vi "ENPH354_LabSCPE_(SubVI).vi"(10 "Save Data":path, 11 "Array":dbl[][](array[numeric])) -> (0 "I_sc [A]":dbl, 1 "I_m [A]":dbl, 2 "V_oc [V]":dbl, 3 "V_m [V]":dbl, 4 "FF":dbl, 5 "R_sh [Ohm]":dbl, 6 "PCE(n)":dbl, 7 "R_s [Ohm]":dbl)   [LabVIEW 2020]
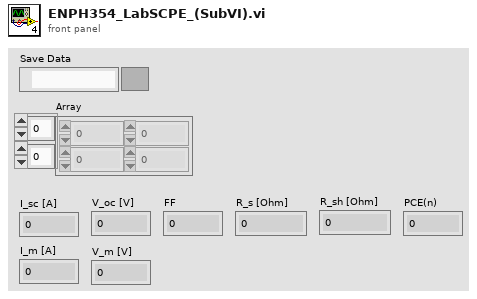
[diagram p1: front panel]
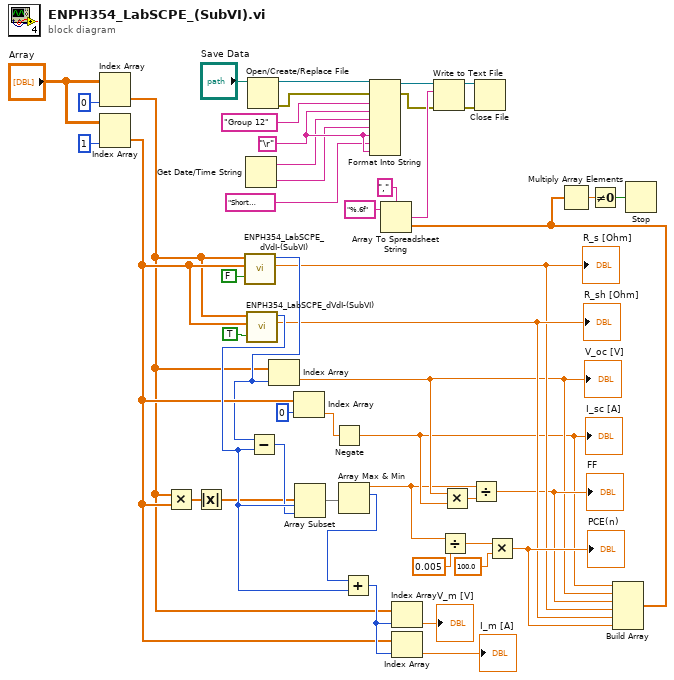
[diagram p0: block diagram]
diagram:
  w20 = "\r"
  n1 = Index Array(array="Array", index (col)=0) -> (element=w27:dbl[])  [unwired: 1 in]
  n2 = Index Array(array="Array", index (col)=1) -> (element=w44:dbl[])  [unwired: 1 in]
  n3 = Multiply(x=w27, y=w44) -> (x*y=w39:dbl[])
  n4 = Absolute Value(x=w39) -> (abs(x)=w40:dbl[])
  n5 = call "ENPH354_LabSCPE_dVdI-(SubVI).vi"("Shunt or Series"=FALSE, "Current in"=w44, "Voltage in"=w27) -> ("dV/dI"=w36:dbl, "IDX"=w41:u8)  [unwired: 7 in]
  "R_s [Ohm]" <- w36
  n6 = Get Date/Time String() -> (date string=w14:string, time string=w15:string)  [unwired: 3 in]
  n7 = call "ENPH354_LabSCPE_dVdI-(SubVI).vi"("Shunt or Series"=TRUE, "Current in"=w44, "Voltage in"=w27) -> ("dV/dI"=w37:dbl, "IDX"=w45:u8)  [unwired: 7 in]
  "R_sh [Ohm]" <- w37
  n8 = Open/Create/Replace File(file path (use dialog)="Save Data") -> (refnum out=w6:refnum<file>, error out=w9:errorcluster)  [unwired: 5 in, 1 out]
  n9 = Subtract(x=w41, y=w45) -> (x-y=w42:u8)
  n10 = Index Array(array=w27, index=w41) -> (element=w34:dbl)
  "V_oc [V]" <- w34
  n11 = Index Array(array=w44, index=0) -> (element=w24:dbl)
  n12 = Array Subset(array=w40, index=w45, length=w42) -> (w43:dbl[])
  n13 = Negate(x=w24) -> (-x=w33:dbl)
  "I_sc [A]" <- w33
  n14 = Array Max & Min(array=w43) -> (max value=w32:dbl, max index (indices)=w46:i32)  [unwired: 2 out]
  n15 = Add(x=w46, y=w45) -> (x+y=w47:i32)
  n16 = Format Into String(initial string=w6, error in=w9, "Group 12" ("input 1"), w20, w14, w15, w20, "Short Circuit Current [A], Open-circuit Voltage [V], Fill Factor, Series Resistance [Ohm], Shunt Resistance [Ohm], Power Conversion Efficiency [%] ", w20) -> (resulting string=w7:refnum<file>, error out=w10:errorcluster)  [unwired: 1 in]
  n17 = Index Array(array=w27, index=w47) -> (element=→"V_m [V]":dbl)
  n18 = Index Array(array=w44, index=w47) -> (element=→"I_m [A]":dbl)
  n19 = Divide(x=w32, y=0.005) -> (x/y=w30:dbl)
  n20 = Multiply(x=w34, y=w33) -> (x*y=w26:dbl)
  n21 = Divide(x=w32, y=w26) -> (x/y=w35:dbl)
  "FF" <- w35
  n22 = Multiply(x=w30, y=100.0) -> (x*y=w38:dbl)
  "PCE(n)" <- w38
  n23 = Build Array(w33, w34, w35, w36, w37, w38) -> (w1:dbl[])
  n24 = Array To Spreadsheet String(delimiter (Tab)=",", array=w1, 3:"%.6f" ("format string")) -> (spreadsheet string=w17:string)
  n25 = Write to Text File(file (use dialog)=w7, text=w17, error in=w10) -> (refnum out=w8:refnum<file>, error out=w11:errorcluster)  [unwired: 1 in, 1 out]
  n26 = Close File(refnum=w8, error in=w11) -> ()  [unwired: 2 out]
  n27 = Multiply Array Elements(1:w1) -> (0:w3:dbl)
  n28 = Not Equal To 0?(x=w3) -> (x != 0?=w2:bool)
  n29 = Stop(stop? (T)=w2) -> ()
